vi "Read DAQ FIFO.vi"(8 "error in (no error)":errorcluster, 9 "Timeout (ms)":i32=100, 10 "Data In":T1[](array[typedef]), 11 "CIFChannels in":refnum<class "CIFChannels.lvclass">) -> (0 "error out":errorcluster, 1 "timed out?":bool, 2 "Data Out":T1[](array[typedef]), 3 "CIFChannels out":refnum<class "CIFChannels.lvclass">, 4 "Header":T2)   [LabVIEW 2021, in "CIFChannels.lvclass"]
uses:
  CIFChannels.lvclass
  CIFChannels.lvclass/CIFChannels.ctl
  CIFCore/Common/CIFCoreCommon.lvlib
  CIFCore/Common/Typedef/Errors.ctl
  ChannelCommon/typedef/FIFO Header.ctl
  ChannelCommon/ChannelCommon.lvlib
  ChannelCommon/typedef/Datatype Waveform.ctl
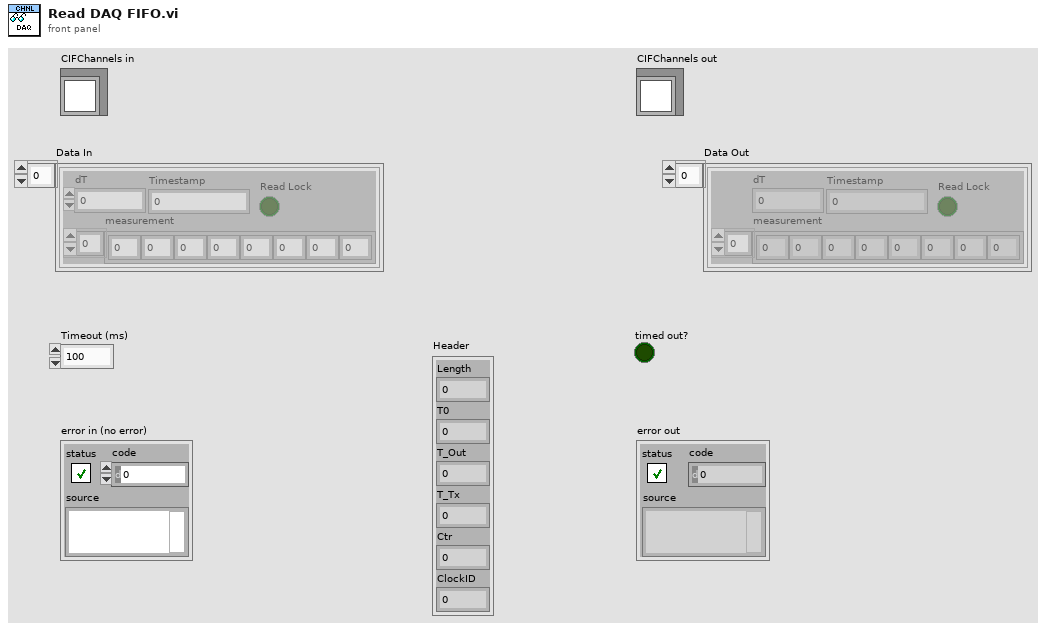
[diagram p1: front panel]
types:
  T1 = typedef "ChannelCommon.lvlib/Datatype Waveform.ctl" = cluster{"measurement":dbl[], "dT":dbl, "Timestamp":u64, "Read Lock":bool}
  T2 = typedef "ChannelCommon.lvlib/FIFO Header.ctl" = cluster{"Length":u64, "T0":u64, "T_Out":u64, "T_Tx":u64, "Ctr":u64, "ClockID":u8}
  T3 = typedef "CIFCoreCommon.lvlib/Errors.ctl" = enum16{"Invalid Clock ID", "Long Sleep", "gRPC Server Not Found", "Config Parse", "Timestamp Wrap", "Delayed Execution", "Duplicate Channel", "Missing Channel", "Incorrect Type", "Flatten Error", "Unflatten Data", "Unique Name", "Plugin Not Found", "Plugin Type Not Found", "Plugin Version Not Found", "Manager Not Found", "Numerical Issue", "Time Jump", "Clock ID Match", "Channel Length"}
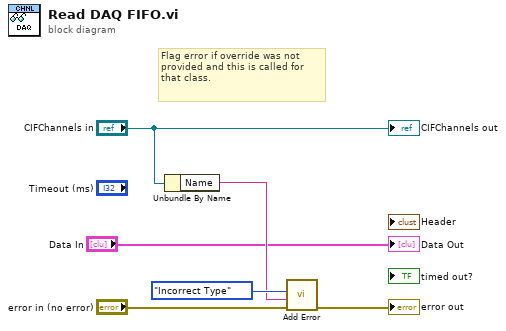
[diagram p0: block diagram]
diagram:
  # "Flag error if override was not provided and this is called for that class."
  n1 = Unbundle By Name("CIFChannels in") -> ("Name"=w2:string)
  n2 = call "Add Error.vi"("error in (no error)"="error in (no error)", "String to Append"=w2, "Error"=Errors."Incorrect Type") -> ("error out"=→"error out":errorcluster)  [unwired: 8 in]
  "CIFChannels out" <- "CIFChannels in"
  "Data Out" <- "Data In"
